vi "2ptderivative.vi"(11 "Counter Value":i32) -> (3 "Numeric":i32)   [LabVIEW 2013]
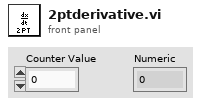
[diagram p1: front panel]
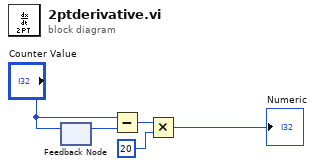
[diagram p0: block diagram]
diagram:
  n1 = feedback #1() -> (w3:i32)  [unwired: 1 in]
  n2 = feedback-in #1("Counter Value") -> ()
  n3 = Subtract(x="Counter Value", y=w3) -> (x-y=w2:i32)
  n4 = Multiply(x=w2, y=20) -> (x*y=→"Numeric":i32)
